vi "Update Plugin Types by Reference.vi"(8 "error in (no error)":errorcluster, 10 "plugin_types":T1[](array[typedef]), 11 "Plugin Types ref in":refnum<vi>) -> (0 "error out":errorcluster, 3 "Plugin Types ref out":refnum<vi>)   [LabVIEW 2021, in "CIF_Manager_UI.lvclass"]
uses:
  CIF_Manager_UI.lvclass
  <vilib>/CIF Foundation/CIF Core/CIFPluginManager/gRPC/CIF_Manager_client/RPC Messages/cif_manager_PluginType.ctl
  <vilib>/CIF Foundation/CIF Core/CIFPluginManager/gRPC/CIF_Manager_client/RPC Messages/cif_common_ShortVersion.ctl
  <vilib>/CIF Foundation/CIF Core/CIFPluginManager/gRPC/CIF_Manager_client/RPC Messages/cif_management_common_PluginMetadata.ctl
  ec76c822-4f10-4c3b-b0a5-b8b1820bcb8b.vi
  <vilib>/Comparison/Less/Less Functor/Less Functor.lvclass
  <vilib>/CIF Foundation/CIF Core/CIFCore/Common/CIFCoreCommon.lvlib
  <vilib>/CIF Foundation/CIF Core/CIFPluginManager/gRPC/CIF_Manager_client/CIF_Manager_client.lvlib
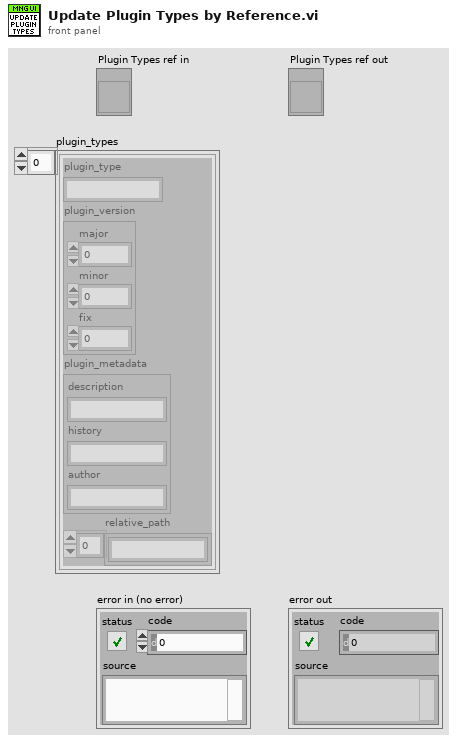
[diagram p1: front panel]
types:
  T1 = typedef "CIF_Manager_client.lvlib/cif_manager_PluginType.ctl" = cluster{"plugin_type":string, "plugin_version":T2, "plugin_metadata":T3, "relative_path":string[]}
  T2 = typedef "CIF_Manager_client.lvlib/cif_common_ShortVersion.ctl" = cluster{"major":u32, "minor":u32, "fix":u32}
  T3 = typedef "CIF_Manager_client.lvlib/cif_management_common_PluginMetadata.ctl" = cluster{"description":string, "history":string, "author":string}
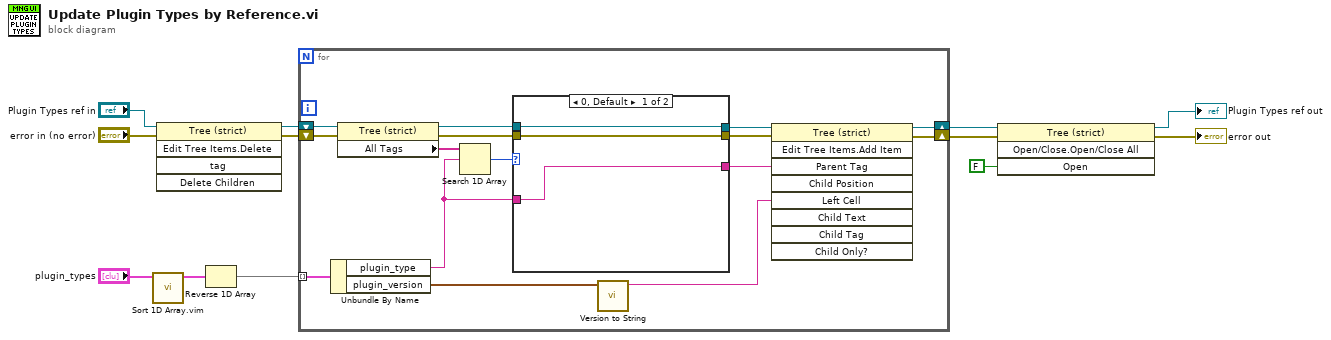
[diagram p0: block diagram]
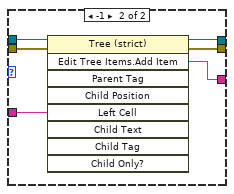
[diagram p2: hidden frame]
diagram:
  n1 = call "Sort 1D Array.vim"("unsorted array"="plugin_types") -> ("sorted array"=w1:T1[])  [unwired: 10 in]
  n2 = invoke class="Tree (strict)" method="Edit Tree Items.Delete"(reference="Plugin Types ref in", error in="error in (no error)") -> (reference out=w11:refnum<vi>, error out=w12:errorcluster)  [unwired: 3 in, 3 out]
  n3 = Reverse 1D Array(array=w1) -> (reversed array=w3:T1[])
  n4 = for {
    tunnel: w3 -> [w24] mode=indexing
    shift-right: [w15] -> w10
    shift-left: w11 -> [w21]
    shift-right: [w26] -> w9
    shift-left: w12 -> [w20]
    n5 = Unbundle By Name(w24) -> ("plugin_type"=w23:string, "plugin_version"=w14:T2)
    n6 = property class="Tree (strict)"(reference=w21, error in=w20) -> (reference out=w17:refnum<vi>, error out=w19:errorcluster, "All Tags"=w18:string[])
    n7 = Search 1D Array(1D array=w18, element=w23) -> (index of element=w22:i32)  [unwired: 1 in]
    n8 = case shown="0, Default" w22 {
      tunnel: [w29 w33] -> w27
      tunnel: [w30 w32] -> w25
      tunnel: w19 -> [w30 w36]
      tunnel: w23 -> [w29 w34]
      tunnel: w17 -> [w28 w35]
      tunnel: [w28 w31] -> w16
      frame 0, Default {
      }
      frame -1 {
        n9 = invoke class="Tree (strict)" method="Edit Tree Items.Add Item"(reference=w35, error in=w36, "Left Cell"=w34) -> (reference out=w31:refnum<vi>, error out=w32:errorcluster, "Edit Tree Items:Add Item"=w33:string)  [unwired: 6 in, 6 out]
      }
    }
    n10 = call <vilib>:"Version to String.vi"("Version"=w14) -> ("Version String"=w13:string)  [unwired: 10 in]
    n11 = invoke class="Tree (strict)" method="Edit Tree Items.Add Item"(reference=w16, error in=w25, "Parent Tag"=w27, "Left Cell"=w13) -> (reference out=w15:refnum<vi>, error out=w26:errorcluster)  [unwired: 5 in, 7 out]
  }
  n12 = invoke class="Tree (strict)" method="Open/Close.Open/Close All"(reference=w10, error in=w9, "Open"=FALSE ("Open?")) -> (reference out=→"Plugin Types ref out":refnum<vi>, error out=→"error out":errorcluster)  [unwired: 1 in, 2 out]
